vi "Enclose in Structure.vi"(6 "Variant in":variant, 7 "Shift Pressed?":bool, 8 "error in":errorcluster, 10 "QD Combo Box Ref":refnum<vi>, 11 "QD Launch VI Ref":refnum<vi>) -> (0 "error out":errorcluster, 4 "Variant out":variant)   [LabVIEW 2020]
doc: "This is merely a Quick Drop shortcut that wires across wires for a flat sequence structure\nThe flat sequence structure is minimally compact, independent of what is drawn.\nThis will surely be replaced once NI enables pass through values to propagate through structures, by default.\n\nDefault Shortcut - [s]"
panel:
  in  "Undo Name":string="Enclose in Structure"
  # "Do not change the connector pane of this VI.\n\nSee the block diagram for directions on how to use this template."
  # "Specify the name of the Undo transaction"
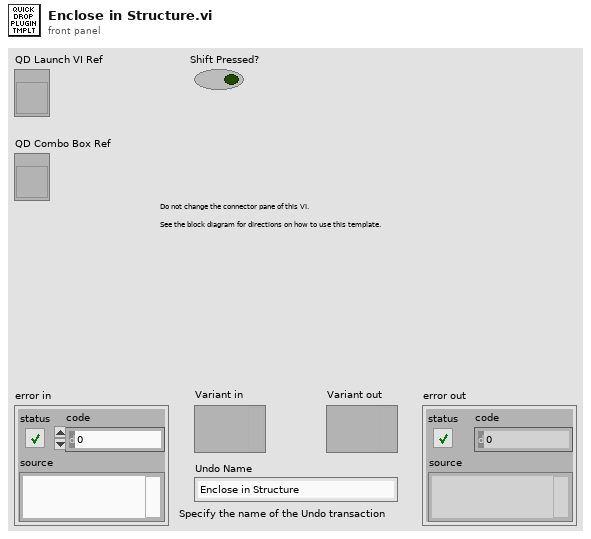
[diagram p1: front panel]
types:
  T1 = typedef "Enclose in Structure - Structure Type.ctl" = enum16{"<Invalid>", "For Loop", "While Loop", "Timed Loop", "Timed Sequence", "Case Structure", "Event Structure", "In Place Element Structure", "Flat Sequence", "Diagram Disable Structure", "Conditional Disable Structure", "Type Specialization Structure"}
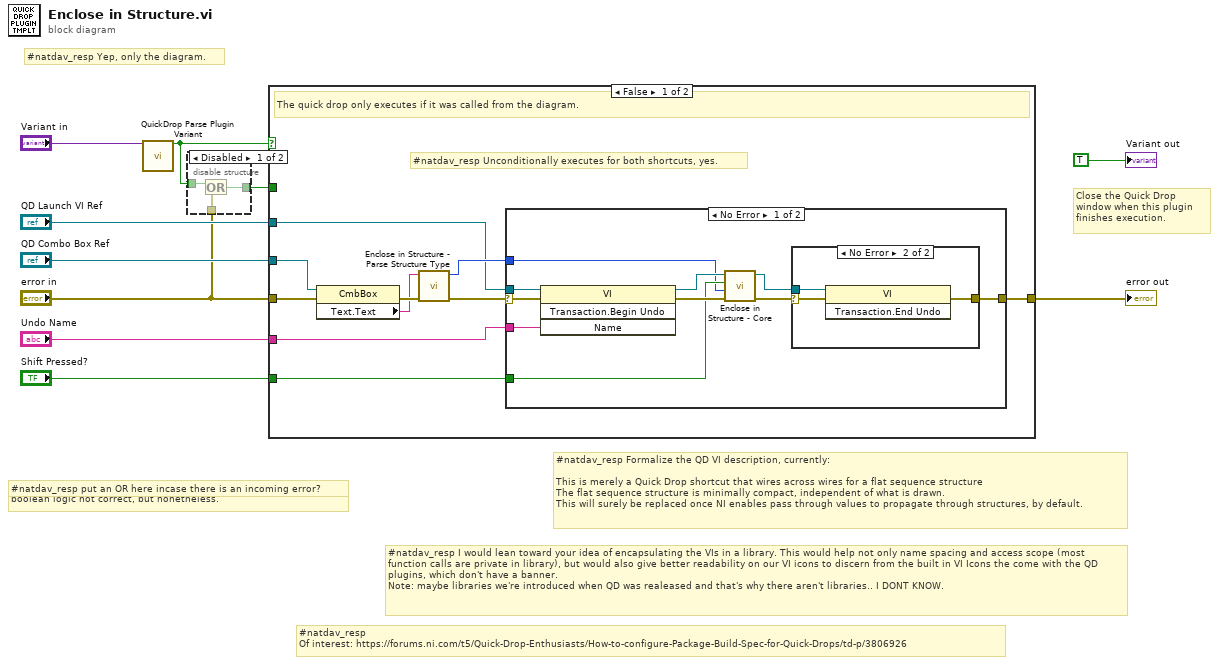
[diagram p0: block diagram]
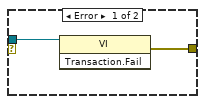
[diagram p3: hidden frame]
diagram:
  # "#natdav_resp\nOf interest: https://forums.ni.com/t5/Quick-Drop-Enthusiasts/How-to-configure-Package-Build-Spec-for-Quick-Drops/td-p/3806926"
  # "#natdav_resp I would lean toward your idea of encapsulating the VIs in a library. This would help not only name spacing and access scope (most function calls are private in library), but would also give better readability on our VI icons to discern from the built in VI Icons the come with the QD plugins, which don't have a banner.\nNote: maybe libraries we're introduced when QD was realeased and that's why there aren't libraries.. I DONT KNOW."
  # "#natdav_resp put an OR here incase there is an incoming error?\nboolean logic not correct, but nonetheless."
  # "#natdav_resp put an OR here incase there is an incoming error?"
  # "#natdav_resp Yep, only the diagram."
  # "#natdav_resp Formalize the QD VI description, currently:\n\nThis is merely a Quick Drop shortcut that wires across wires for a flat sequence structure\nThe flat sequence structure is minimally compact, independent of what is drawn.\nThis will surely be replaced once NI enables pass through values to propagate through structures, by default."
  # "Close the Quick Drop window when this plugin finishes execution."
  n1 = call <vilib>:"QuickDrop Parse Plugin Variant.vi"("QDKS Variant in"="Variant in") -> ("QD Launch VI Panel?"=w3:bool)  [unwired: 12 in, 2 out]
  n2 = disable-structure shown="Disabled" {
    disable-tunnel: w3 -> [w13 _]
    disable-tunnel: "error in" -> [w12 _]
    disable-tunnel: [w11 _] -> w1
    frame Disabled {
      n3 = Or(x=w13, y=w12) -> (x .or. y?=w11:bool)
    }
    frame Enabled {
    }
  }
  n4 = case shown="False" w3 {
    tunnel: "error in" -> [w21 w40]
    tunnel: [w23 w40] -> w7
    tunnel: "QD Launch VI Ref" -> [w14 _]
    tunnel: "Undo Name" -> [w22 _]
    tunnel: "QD Combo Box Ref" -> [w20 _]
    tunnel: "Shift Pressed?" -> [w19 _]
    tunnel: w1 -> [_ _]
    frame False {
      # "#natdav_resp Unconditionally executes for both shortcuts, yes."
      # "The quick drop only executes if it was called from the diagram."
      n5 = property class="CmbBox"(reference=w20, error in=w21) -> (error out=w18:errorcluster, "Text.Text"=w16:string)  [unwired: 1 out]
      n6 = call "Enclose in Structure - Parse Structure Type.vi"("error in"=w18, "QD Text"=w16) -> ("error out"=w17:errorcluster, "Structure Type"=w15:T1)  [unwired: 8 in]
      n7 = case shown="No Error" w17 {
        selector: w17 -> [w26 w39]
        tunnel: [w33 w39] -> w23
        tunnel: w22 -> [w32 _]
        tunnel: w19 -> [w27 _]
        tunnel: w15 -> [w25 _]
        tunnel: w14 -> [w24 _]
        frame No Error {
          n8 = invoke class="VI" method="Transaction.Begin Undo"(reference=w24, error in=w26, "Name"=w32) -> (reference out=w30:refnum<vi>, error out=w31:errorcluster)  [unwired: 1 in, 2 out]
          n9 = call "Enclose in Structure - Core.vi"("error in"=w31, "Structure Type"=w25, "T: Replace / F: Enclose"=w27, "VI in"=w30) -> ("error out"=w29:errorcluster, "VI out"=w28:refnum<vi>)  [unwired: 6 in]
          n10 = case shown="No Error" w29 {
            selector: w29 -> [_ w36]
            tunnel: w28 -> [w34 w37]
            tunnel: [w35 w38] -> w33
            frame Error {
              n11 = invoke class="VI" method="Transaction.Fail"(reference=w34) -> (error out=w35:errorcluster)  [unwired: 2 in, 2 out]
            }
            frame No Error {
              n12 = invoke class="VI" method="Transaction.End Undo"(reference=w37, error in=w36) -> (error out=w38:errorcluster)  [unwired: 1 in, 2 out]
            }
          }
        }
        frame Error {
        }
      }
    }
    frame True {
    }
  }
  "error out" <- w7
  "Variant out" <- TRUE
